vi "CalcRTUncertainty.vi"(9 "Limits":dbl[][](array[numeric]), 10 "Uncertainties":dbl[][](array[numeric]), 11 "Step Data":dbl[][][](array[numeric])) -> (2 "Uncert":dbl[][][](array[numeric]), 3 "Range":dbl[][][](array[numeric]))   [LabVIEW 2014]
panel:
  out "Waveform Graph":dbl[](graph)
  out "Phase":i32
  # "VA                      VB                     VC                     V+                     IA                         IB                    IC                            I+                  Freq                    ROCOF"
  # "RT + unc\n\nRT\n\nRT - unc"
  # "VA                      VB                     VC                     V+                     IA                         IB                    IC                            I+                  Freq                    ROCOF"
  # "plus\n\nRT\n\nminus"
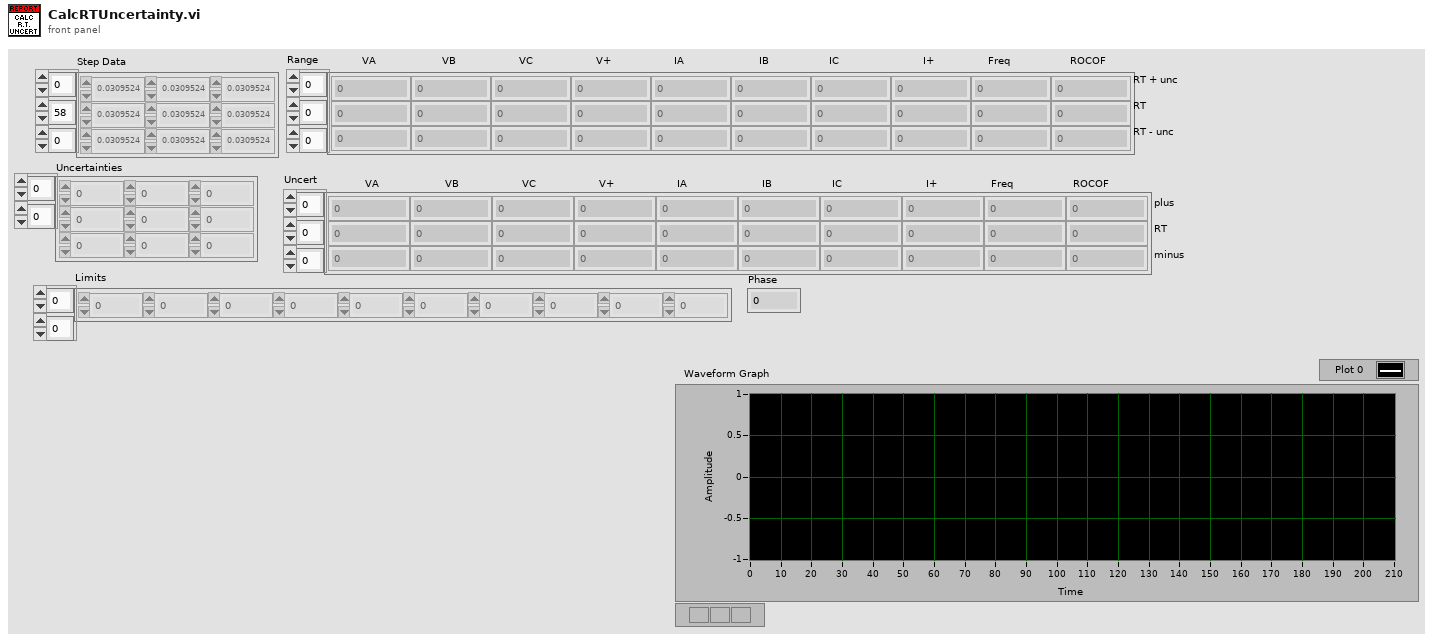
[diagram p1: front panel]
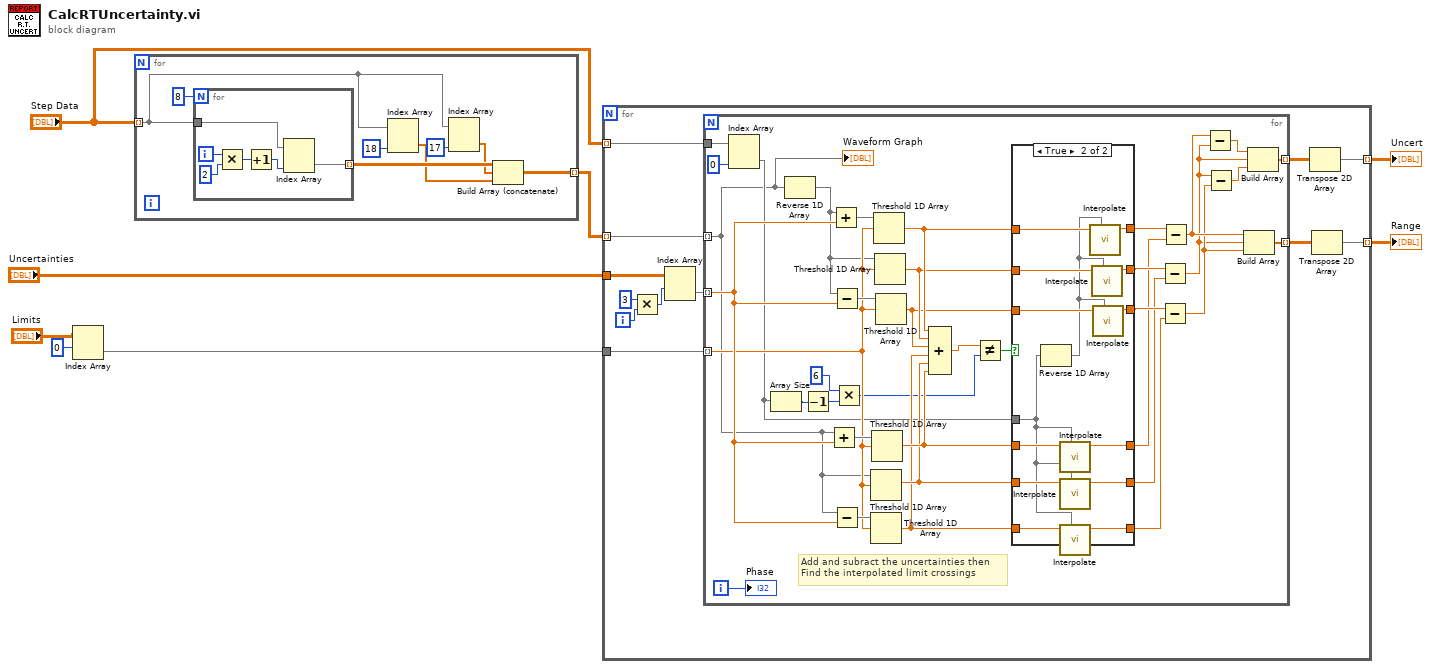
[diagram p0: block diagram]
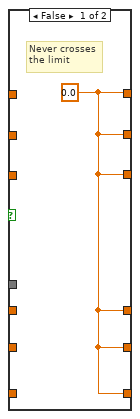
[diagram p2: hidden frame]
diagram:
  n1 = Index Array(array="Limits", index (row)=0) -> (element=w1:dbl[])  [unwired: 1 in]
  n2 = for {
    tunnel: "Step Data" -> [w14] mode=indexing
    tunnel: [w9] -> w5 mode=indexing
    n3 = for {
      N: 8 -> [_]
      tunnel: w14 -> [w19]
      tunnel: [w17] -> w16 mode=indexing
      i -> [w22]
      n4 = Multiply(x=w22, y=2) -> (x*y=w20:i32)
      n5 = Increment(x=w20) -> (x+1=w18:i32)
      n6 = Index Array(array=w19, index (col)=w18) -> (element=w17:dbl[])  [unwired: 1 in]
    }
    n7 = Index Array(array=w14, index (col)=18 ("disabled index (col)")) -> (element=w11:dbl[])  [unwired: 1 in]
    n8 = Index Array(array=w14, index (col)=17 ("disabled index (col)")) -> (element=w10:dbl[])  [unwired: 1 in]
    n9 = Build Array (concatenate)(w16, w10, w11) -> (w9:dbl[][])
  }
  n10 = for {
    tunnel: w5 -> [w34] mode=indexing
    tunnel: "Uncertainties" -> [w24]
    tunnel: w1 -> [w33]
    tunnel: "Step Data" -> [w32] mode=indexing
    tunnel: [w30] -> w6 mode=indexing
    tunnel: [w28] -> w7 mode=indexing
    i -> [w27]
    n11 = Multiply(x=3, y=w27) -> (x*y=w26:i32)
    n12 = Index Array(array=w24, index (row)=w26) -> (element=w23:dbl[])  [unwired: 1 in]
    n13 = for {
      tunnel: w34 -> [w35] mode=indexing
      tunnel: w23 -> [w66] mode=indexing
      tunnel: w33 -> [w64] mode=indexing
      tunnel: w32 -> [w70]
      tunnel: [w56] -> w31 mode=indexing
      tunnel: [w50] -> w29 mode=indexing
      i -> [w49]
      # "Add and subract the uncertainties then\nFind the interpolated limit crossings"
      n14 = Index Array(array=w70, index (col)=0 ("disabled index (col)")) -> (element=w42:dbl[])  [unwired: 1 in]
      n15 = Array Size(array=w42) -> (size(s)=w37:i32)
      n16 = Reverse 1D Array(array=w35) -> (reversed array=w63:dbl[])
      n17 = Decrement(x=w37) -> (x-1=w36:i32)
      n18 = Add(x=w35, y=w66) -> (x+y=w67:dbl[])
      n19 = Add(x=w63, y=w66) -> (x+y=w68:dbl[])
      n20 = Subtract(x=w63, y=w66) -> (x-y=w71:dbl[])
      n21 = Subtract(x=w35, y=w66) -> (x-y=w65:dbl[])
      n22 = Multiply(x=6, y=w36) -> (x*y=w39:i32)
      n23 = Threshold 1D Array(2:w64, 3:w35) -> (0:w44:dbl)  [unwired: 1 in]
      n24 = Threshold 1D Array(2:w64, 3:w65) -> (0:w43:dbl)  [unwired: 1 in]
      n25 = Threshold 1D Array(2:w64, 3:w67) -> (0:w45:dbl)  [unwired: 1 in]
      n26 = Threshold 1D Array(2:w64, 3:w68) -> (0:w48:dbl)  [unwired: 1 in]
      n27 = Threshold 1D Array(2:w64, 3:w63) -> (0:w47:dbl)  [unwired: 1 in]
      n28 = Threshold 1D Array(2:w64, 3:w71) -> (0:w46:dbl)  [unwired: 1 in]
      n29 = Compound Arithmetic op=ADD(w48, w47, w46, w43, w44, w45) -> (w40:dbl)
      n30 = Not Equal?(x=w40, y=w39) -> (x != y?=w41:bool)
      n31 = case shown="True" w41 {
        tunnel: w48 -> [_ w86]
        tunnel: w47 -> [_ w85]
        tunnel: w46 -> [_ w84]
        tunnel: w45 -> [_ w83]
        tunnel: w44 -> [_ w82]
        tunnel: w43 -> [_ w81]
        tunnel: [w72 w79] -> w62
        tunnel: [w72 w78] -> w61
        tunnel: [w72 w77] -> w60
        tunnel: [w72 w76] -> w59
        tunnel: [w72 w75] -> w58
        tunnel: [w72 w74] -> w57
        tunnel: w42 -> [_ w73]
        frame False {
          w72 = 0.0
          # "Never crosses\nthe limit"
        }
        frame True {
          n32 = Reverse 1D Array(array=w73) -> (reversed array=w80:dbl[])
          n33 = call "Interpolate.vi"("Array"=w73, "Index"=w83) -> ("Value"=w76:dbl)  [unwired: 9 in]
          n34 = call "Interpolate.vi"("Array"=w73, "Index"=w82) -> ("Value"=w75:dbl)  [unwired: 9 in]
          n35 = call "Interpolate.vi"("Array"=w73, "Index"=w81) -> ("Value"=w74:dbl)  [unwired: 9 in]
          n36 = call "Interpolate.vi"("Array"=w80, "Index"=w86) -> ("Value"=w79:dbl)  [unwired: 9 in]
          n37 = call "Interpolate.vi"("Array"=w80, "Index"=w85) -> ("Value"=w78:dbl)  [unwired: 9 in]
          n38 = call "Interpolate.vi"("Array"=w80, "Index"=w84) -> ("Value"=w77:dbl)  [unwired: 9 in]
        }
      }
      n39 = Subtract(x=w61, y=w58) -> (x-y=w51:dbl)
      n40 = Subtract(x=w60, y=w57) -> (x-y=w54:dbl)
      n41 = Subtract(x=w62, y=w59) -> (x-y=w55:dbl)
      n42 = Subtract(x=w55, y=w51) -> (x-y=w53:dbl)
      n43 = Subtract(x=w51, y=w54) -> (x-y=w52:dbl)
      n44 = Build Array(w55, w51, w54) -> (w56:dbl[])
      n45 = Build Array(w53, w51, w52) -> (w50:dbl[])
      "Phase" <- w49
      "Waveform Graph" <- w35
    }
    n46 = Transpose 2D Array(2D array=w29) -> (transposed array=w28:dbl[][])
    n47 = Transpose 2D Array(2D array=w31) -> (transposed array=w30:dbl[][])
  }
  "Uncert" <- w7
  "Range" <- w6
